vi "wait_for_psexec.vi"(10 "error out":errorcluster, 11 "base path":path) -> (3 "error out 2":errorcluster)   [LabVIEW 2018]
panel:
  out "appended path":path
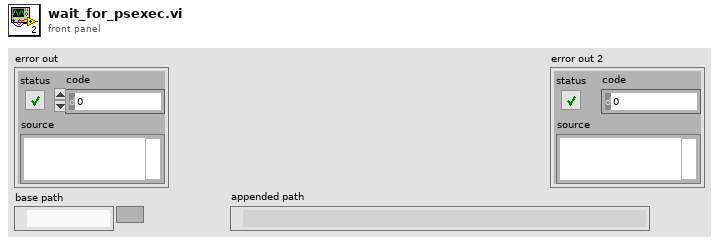
[diagram p1: front panel]
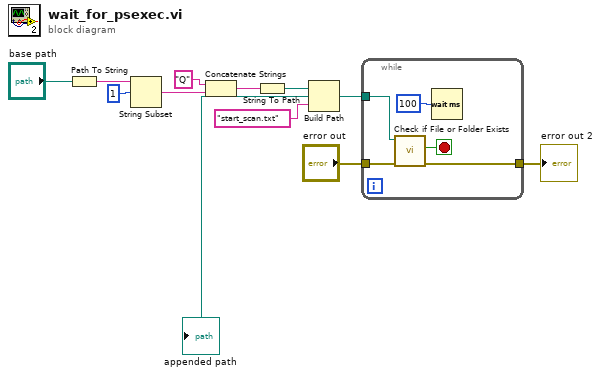
[diagram p0: block diagram]
diagram:
  n1 = Path To String(path="base path") -> (string=w6:string)
  n2 = String Subset(string=w6, offset (0)=1) -> (substring=w3:string)  [unwired: 1 in]
  n3 = Concatenate Strings("Q" ("string"), w3) -> (w2:string)
  n4 = String To Path(string=w2) -> (path=w1:path)
  n5 = Build Path(base path=w1, name or relative path="start_scan.txt") -> (appended path=w11:path)
  "appended path" <- w11
  n6 = while {
    tunnel: "error out" -> [w14]
    tunnel: [w13] -> w8
    tunnel: w11 -> [w12]
    stop <- w16 stop-if-true
    n7 = call <vilib>:"Check if File or Folder Exists.vi"("error in (no error)"=w14, "path"=w12) -> ("error out"=w13:errorcluster, "file or folder exists?"=w16:bool)  [unwired: 7 in, 1 out]
    n8 = Wait (ms)(milliseconds to wait=u32 100) -> ()  [unwired: 1 out]
  }
  "error out 2" <- w8
